vi "MES_Base_ConfigFP.vi"(0 "reference in":refnum<class "MES_Base.lvclass">, 5 "error in (no error)":errorcluster) -> (14 "reference out":refnum<class "MES_Base.lvclass">, 19 "error out":errorcluster)   [LabVIEW 2022 SP3, in "MES_Base.lvlib" / "MES_Base.lvclass"]
uses:
  MES_Base.lvclass
  protected/Config.ctl
  Components/ViPER.lvlibp/ViPER.lvclass
  C:/Projects/Medulla/ViPER/Examples/Flux_Capacitor_Tester/Components/ViPER.lvlibp/ViPER.lvclass
panel:
  in  "Config":T1
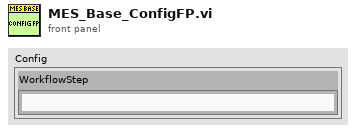
[diagram p1: front panel]
types:
  T1 = typedef "MES_Base.lvlib/MES_Base.lvclass/Config.ctl" = cluster{"WorkflowStep":string}
  T2 = enum32{"Invalid", "Standard", "Closed", "Hidden", "Minimized", "Maximized"}
  T3 = typedef "MES_Base.lvlib/MES_Base.lvclass/ObjectAttributes.ctl" = cluster{"Config":T1}
  T4 = typedef "LVRectTypeDef.ctl" = cluster{"Left":i16, "Top":i16, "Right":i16, "Bottom":i16}
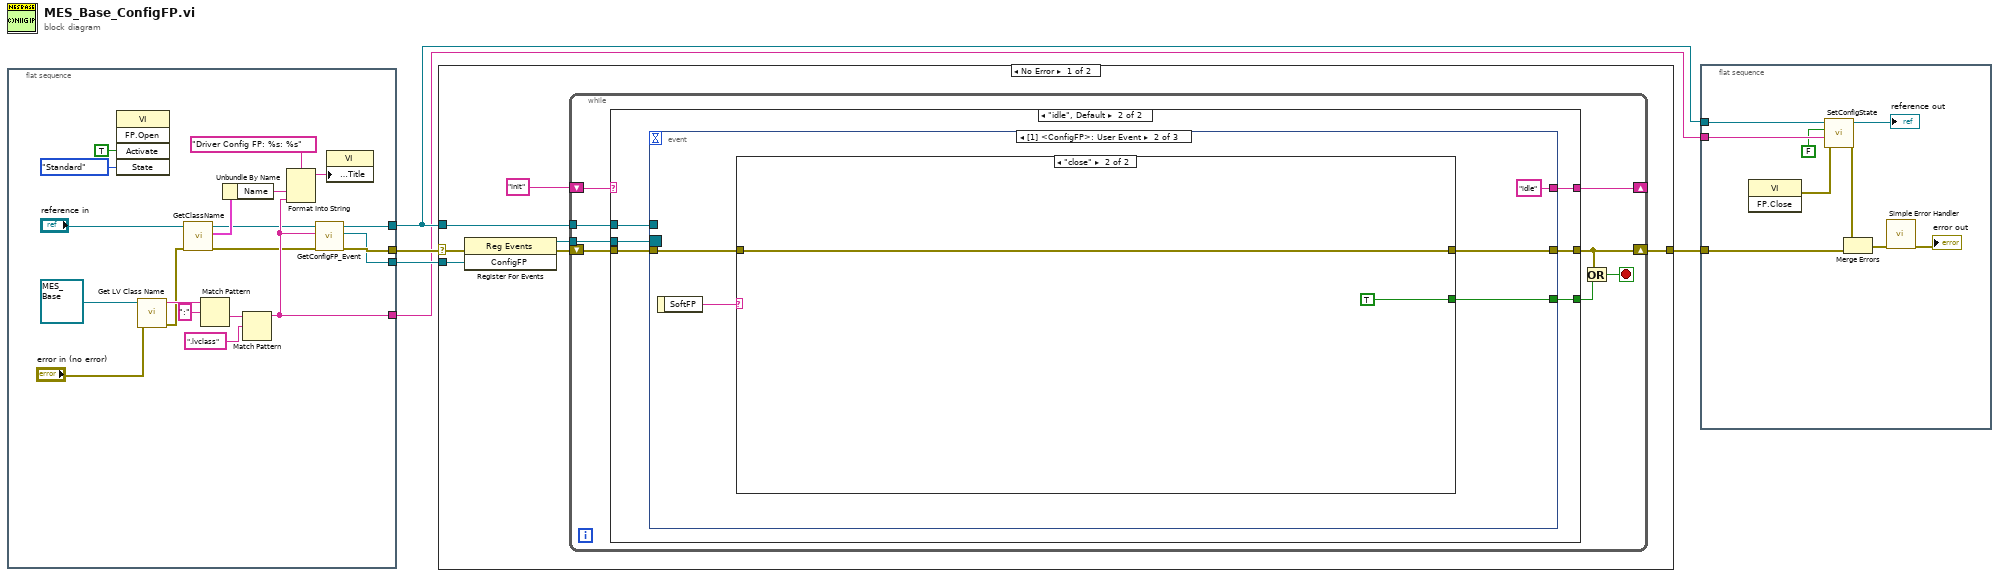
[diagram p0: block diagram]
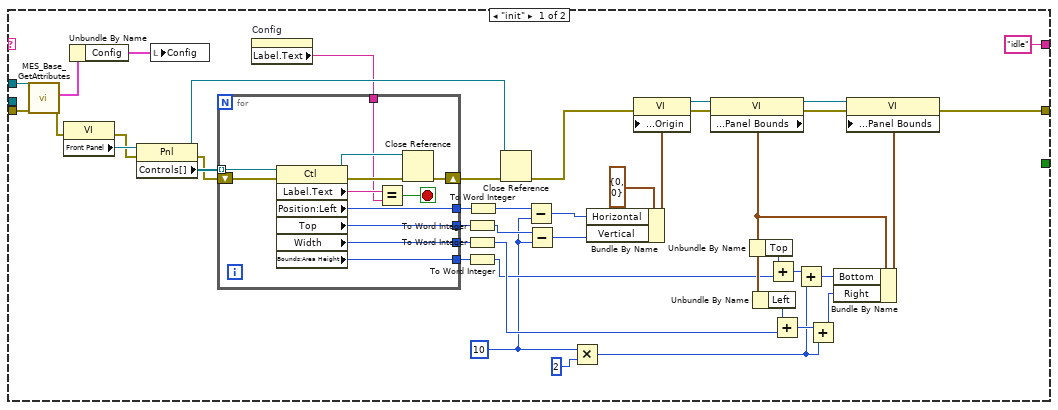
[diagram p2: hidden frame]
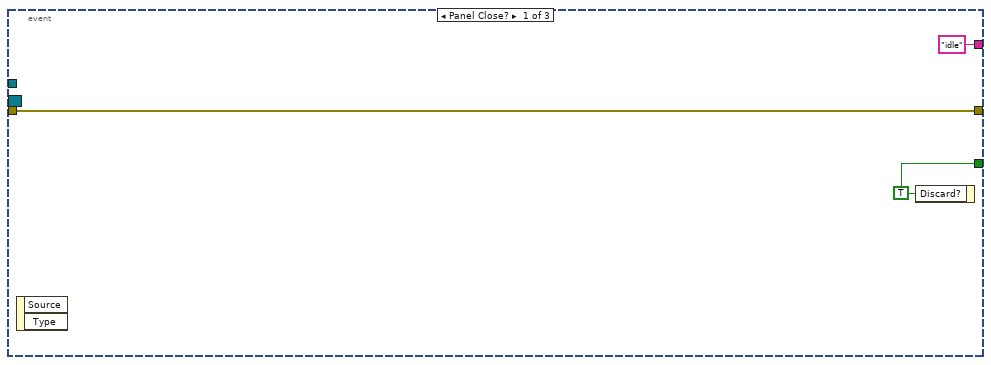
[diagram p3: hidden frame]
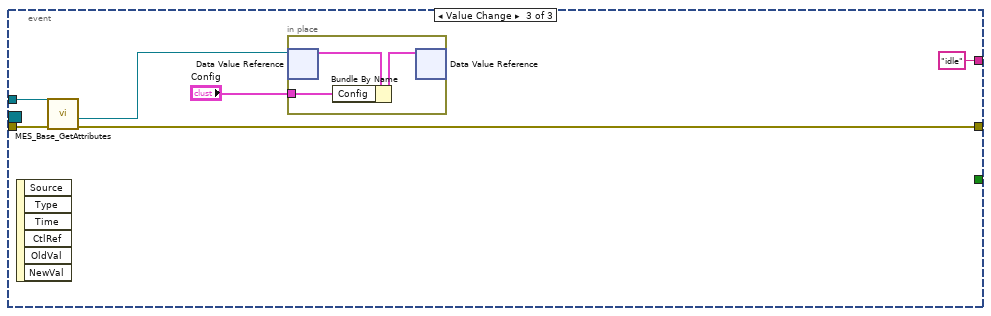
[diagram p5: hidden frame]
diagram:
  n1 = flat-sequence {
    tunnel: [w21] -> w5
    tunnel: [w22] -> w2
    tunnel: [w20] -> w3
    tunnel: [w12] -> w1
    frame #0 {
      n2 = invoke class="VI" method="FP.Open"("Activate"=TRUE ("Activate?"), "State"=T2."Standard") -> ()  [unwired: 3 in, 5 out]
      n3 = call <vilib>:"Get LV Class Name.vi"("error in (no error)"="error in (no error)", "object"=refnum<class "MES_Base.lvclass"> refnum ("reference")) -> ("error out"=w10:errorcluster, "class name"=w18:string)  [unwired: 8 in]
      n4 = call "GetClassName.vi"("error in (no error)"=w10, "reference in"="reference in") -> ("error out"=w8:errorcluster, "Details"=w7:cluster{"Name":string, "Class":string}, "reference out"=w6:refnum<class "MES_Base.lvclass">)  [unwired: 7 in]
      n5 = Match Pattern(string=w18, regular expression=":") -> (after substring=w17:string)  [unwired: 1 in, 3 out]
      n6 = Unbundle By Name(w7) -> ("Name"=w23:string)
      n7 = Match Pattern(string=w17, regular expression=".lvclass") -> (before substring=w12:string)  [unwired: 1 in, 3 out]
      n8 = Format Into String(format string="Driver Config FP: %s: %s", w23, w12) -> (resulting string=w25:string)  [unwired: 2 in, 1 out]
      n9 = call-dynamic "GetConfigFP_Event.vi"("error in (no error)"=w8, "Ancestor"=w12, "reference in"=w6) -> ("error out"=w21:errorcluster, "ConfigFP"=w20:refnum<user-event>, "reference out"=w22:refnum<class "MES_Base.lvclass">)  [unwired: 6 in]
      n10 = property class="VI"("Front Panel.Title"=w25) -> ()  [unwired: 2 in, 2 out]
    }
  }
  n11 = case shown="No Error" w5 {
    selector: w5 -> [w30 w121]
    tunnel: [w26 w121] -> w4
    tunnel: w2 -> [w27 _]
    tunnel: w3 -> [w32 _]
    frame No Error {
      n12 = register-events(error in=w30, w32) -> (reference out=w31:refnum<event-registration>, error out=w29:errorcluster)  [unwired: 1 in]
      n13 = while {
        shift-right: [w37] -> w26
        shift-left: w29 -> [w40]
        tunnel: w31 -> [w39]
        tunnel: w27 -> [w38]
        shift-right: [w33] -> _
        shift-left: "init" -> [w34]
        stop <- w36 stop-if-true
        n14 = case shown="\"idle\", Default" w34 {
          tunnel: w40 -> [w81 w100]
          tunnel: w39 -> [_ w99]
          tunnel: w38 -> [w80 w98]
          tunnel: [w43 w97] -> w37
          tunnel: [_ w96] -> w35
          tunnel: ["idle" w95] -> w33
          frame "init" {
            w45 = i16 10 ("16bit integer")
            n15 = call "MES_Base_GetAttributes.vi"("error in (no error)"=w81, "reference in"=w80) -> ("error out"=w44:errorcluster, "Data"=w79:T3)  [unwired: 6 in, 2 out]
            n16 = property on="Property Node" class="VI"(error in=w44) -> (error out=w75:errorcluster, "Front Panel"=w77:refnum<vi>)  [unwired: 1 in, 1 out]
            n17 = Unbundle By Name(w79) -> ("Config"=w78:T1)
            n18 = property on="Property Node" class="Pnl"(reference=w77, error in=w75) -> (reference out=w50:refnum<vi>, error out=w74:errorcluster, "Controls[]"=w76:refnum<vi>[])
            n19 = local write "Config"(w78) -> ()
            n20 = property on="Config" class="Clust (strict)"() -> ("Label.Text"=w41:string)  [unwired: 2 in, 2 out]
            n21 = for {
              tunnel: w76 -> [w94] mode=indexing
              tunnel: [w90] -> w49
              tunnel: [w89] -> w47
              tunnel: [w88] -> w46
              shift-right: [w85] -> w51
              shift-left: w74 -> [w91]
              tunnel: [w87] -> w48
              tunnel: w41 -> [w83]
              stop <- w92 stop-if-true
              n22 = property class="Ctl"(reference=w94, error in=w91) -> (reference out=w84:refnum<vi>, error out=w86:errorcluster, "Label.Text"=w93:string, "Position:Left"=w90:i32, "Top"=w87:i32, "Width"=w89:u32, "Bounds:Area Height"=w88:u32)
              n23 = Equal?(x=w93, y=w83) -> (x = y?=w92:bool)
              n24 = Close Reference(reference=w84, error in (no error)=w86) -> (error out=w85:errorcluster)
            }
            n25 = To Word Integer(number=w48) -> (16bit integer=w52:i16)
            n26 = To Word Integer(number=w47) -> (16bit integer=w55:i16)
            n27 = To Word Integer(number=w46) -> (16bit integer=w54:i16)
            n28 = To Word Integer(number=w49) -> (16bit integer=w53:i16)
            n29 = Close Reference(reference=w50, error in (no error)=w51) -> (error out=w42:errorcluster)
            n30 = Subtract(x=w53, y=w45) -> (x-y=w62:i16)
            n31 = Subtract(x=w52, y=w45) -> (x-y=w63:i16)
            n32 = Multiply(x=w45, y=i16 2) -> (x*y=w56:i16)
            n33 = Bundle By Name(cluster=cluster{"Horizontal":i16, "Vertical":i16} {"Horizontal"=0, "Vertical"=0} ("Front Panel Window:Origin"), "Horizontal"=w62, "Vertical"=w63) -> (w60:cluster{"Horizontal":i16, "Vertical":i16})
            n34 = property on="Property Node" class="VI"(error in=w42, "Front Panel Window:Origin"=w60) -> (reference out=w72:refnum<vi>, error out=w58:errorcluster)  [unwired: 1 in]
            n35 = property on="Property Node" class="VI"(reference=w72, error in=w58) -> (reference out=w73:refnum<vi>, error out=w57:errorcluster, "Front Panel Window:Panel Bounds"=w64:T4)
            n36 = Unbundle By Name(w64) -> ("Top"=w65:i16)
            n37 = Unbundle By Name(w64) -> ("Left"=w66:i16)
            n38 = Add(x=w65, y=w54) -> (x+y=w70:i16)
            n39 = Add(x=w66, y=w55) -> (x+y=w68:i16)
            n40 = Add(x=w70, y=w56) -> (x+y=w71:i16)
            n41 = Add(x=w68, y=w56) -> (x+y=w69:i16)
            n42 = Bundle By Name(cluster=w64, "Bottom"=w71, "Right"=w69) -> (w67:T4)
            n43 = property on="Property Node" class="VI"(reference=w73, error in=w57, "Front Panel Window:Panel Bounds"=w67) -> (error out=w43:errorcluster)  [unwired: 1 out]
          }
          frame "idle", Default {
            n44 = event shown="[1] <ConfigFP>: User Event" {
              selector: w99 -> [_ _ _]
              dyn-events: _ -> [_ _ _]
              timeout: _ -> [_ _ _]
              tunnel: w100 -> [w103 w108 w117]
              tunnel: [w103 w106 w114] -> w97
              tunnel: [w102 w105 _] -> w96
              tunnel: w98 -> [_ _ w116]
              tunnel: ["idle" "idle" "idle"] -> w95
              event Panel Close? {
                w102 = TRUE ("Discard?")
                n45 = event-data() -> ()  [unwired: 1 in, 2 out]
                n46 = event-data("Discard?"=w102) -> ()  [unwired: 1 in, 1 out]
              }
              event User Event {
                n47 = event-data() -> ("SoftFP"=w107:string)  [unwired: 1 in]
                n48 = case shown="\"close\"" w107 {
                  tunnel: w108 -> [w109 w111]
                  tunnel: [w109 w111] -> w106
                  tunnel: [_ TRUE ("Discard?")] -> w105
                  frame Default {
                  }
                  frame "close" {
                  }
                }
              }
              event Value Change {
                n49 = event-data() -> ()  [unwired: 1 in, 6 out]
                n50 = call "MES_Base_GetAttributes.vi"("error in (no error)"=w117, "reference in"=w116) -> ("error out"=w114:errorcluster, "DataRef"=w115:refnum<data-value>)  [unwired: 6 in, 2 out]
                n51 = in-place {
                  in-place-border: "Config" -> [w118]
                  n52 = in-place-dvr #1(w115) -> (w120:T3)  [unwired: 1 out]
                  n53 = Bundle By Name(cluster=w120, "Config"=w118) -> (w119:T3)
                  n54 = in-place-dvr #1(w119) -> ()  [unwired: 2 out]
                }
              }
            }
          }
        }
        n55 = Or(x=w37, y=w35) -> (x .or. y?=w36:bool)
      }
    }
    frame Error {
    }
  }
  n56 = flat-sequence {
    tunnel: w4 -> [w128]
    tunnel: w2 -> [w124]
    tunnel: w1 -> [w126]
    frame #0 {
      n57 = invoke class="VI" method="FP.Close"() -> (error out=w127:errorcluster)  [unwired: 3 in, 2 out]
      n58 = call "SetConfigState.vi"("error in (no error)"=w127, "Ancestor"=w126, "Config Open"=FALSE ("SP Open"), "reference in"=w124) -> ("error out"=w122:errorcluster, "reference out"=→"reference out":refnum<class "MES_Base.lvclass">)  [unwired: 6 in]
      n59 = Merge Errors(w122, w128) -> (w130:errorcluster)
      n60 = call <vilib>:"Simple Error Handler.vi"("error in (no error)"=w130) -> ("error out"=→"error out":errorcluster)  [unwired: 4 in, 4 out]
    }
  }
